vi "Unit Test.vi"() -> ()   [LabVIEW 2019, in "UIs.lvlib"]
uses:
  UIs.lvlib
  User Event/Controls/UE Abort Action.ctl
  Image/Image.lvlib
  Camera/Andor/Andor.lvlib
  Laser/Coherent/Coherent.lvlib
  LED/LED.lvlib
  Motion/Allmotion/Allmotion.lvlib
  Initialize/Initialize.lvlib
panel:
  in  "Laser":bool
  out "Motion":bool
  out "LED":bool
  out "Laser":bool
  out "Camera":bool
  in  "Open":bool
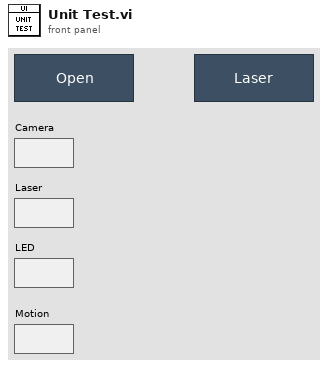
[diagram p1: front panel]
types:
  T1 = typedef "UE Abort Action.ctl" = enum16{"Create", "Get", "Destroy"}
  T2 = typedef "Andor.lvlib/SEQ Data.ctl" = cluster{"Initialize Sucess?":bool, "Image Ref":T3, "VI Refnum":refnum<vi>}
  T3 = typedef "IMAQ Image.ctl" = refnum<image>
  T4 = typedef "Coherent.lvlib/SEQ Data.ctl" = cluster{"Initialize Success?":bool, "VI Refnum":refnum<vi>}
  T5 = typedef "LED.lvlib/SEQ Data.ctl" = cluster{"Initialize Sucess?":bool, "BL2 Regulator":dbl, "BL1 Regulator":dbl, "Blood Sensor 1":dbl, "Blood Sensor 2":dbl, "Air Pressure Sensor":dbl, "Force Snesor 1":u32, "Force Snesor 2":u32, "VI Refnum":refnum<vi>}
  T6 = typedef "Allmotion.lvlib/SEQ Data.ctl" = cluster{"Position":i32[], "Arrived?":bool, "VISA name":refnum<visa-resource-name>, "Initialize Done?":bool, "State":string, "VI Refnum":refnum<vi>, "Dichroic Position":string[]}
  T7 = typedef "Initialize.lvlib/SEQ Data.ctl" = cluster{"Folder Path":path}
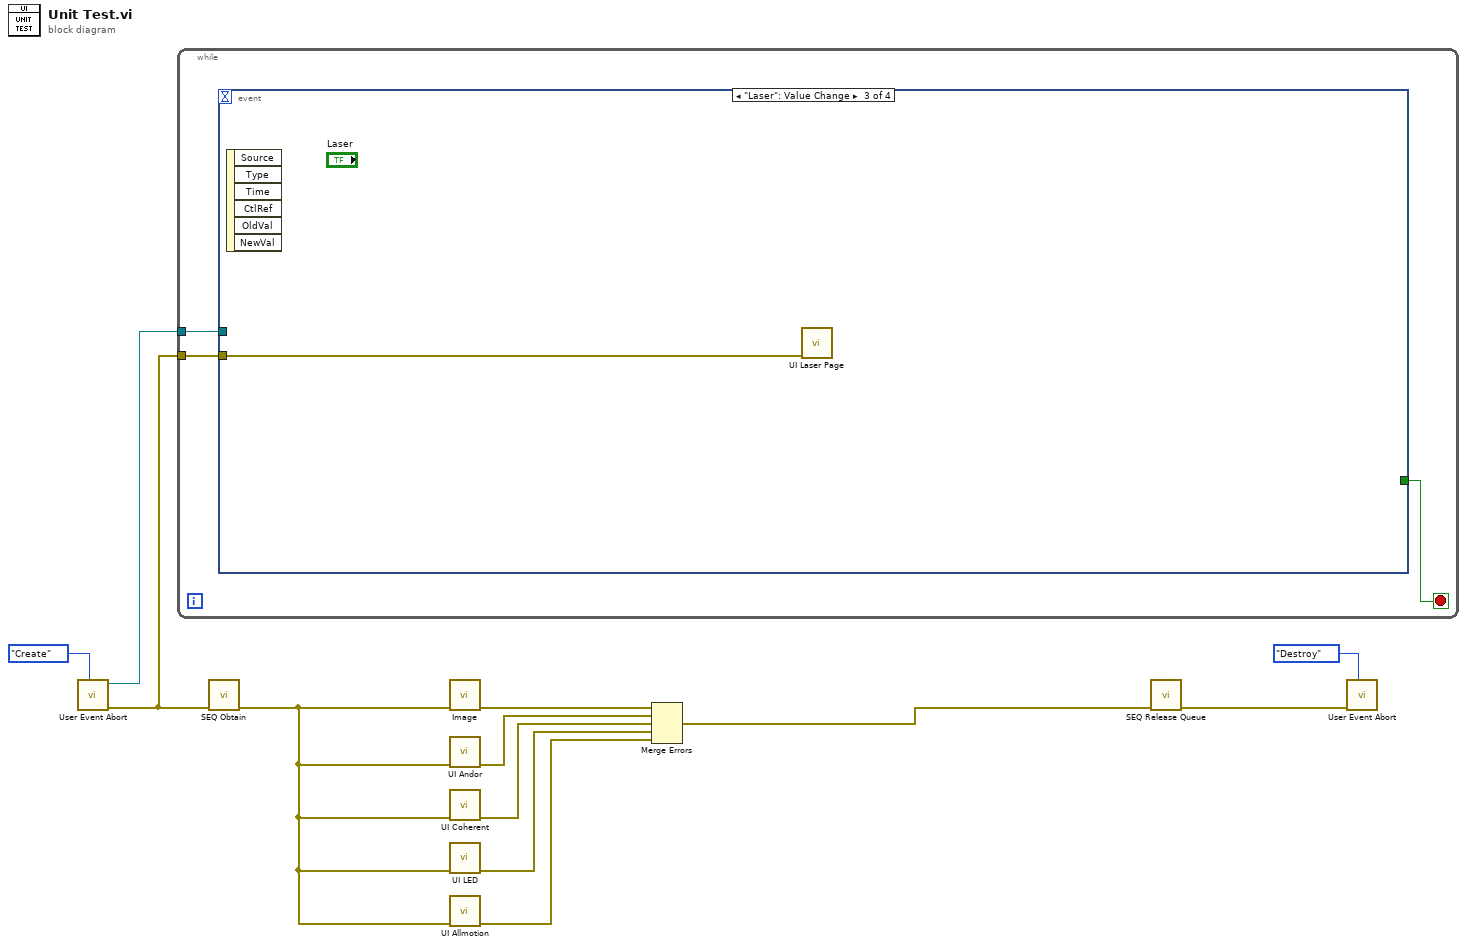
[diagram p0: block diagram]
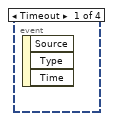
[diagram p2: hidden frame]
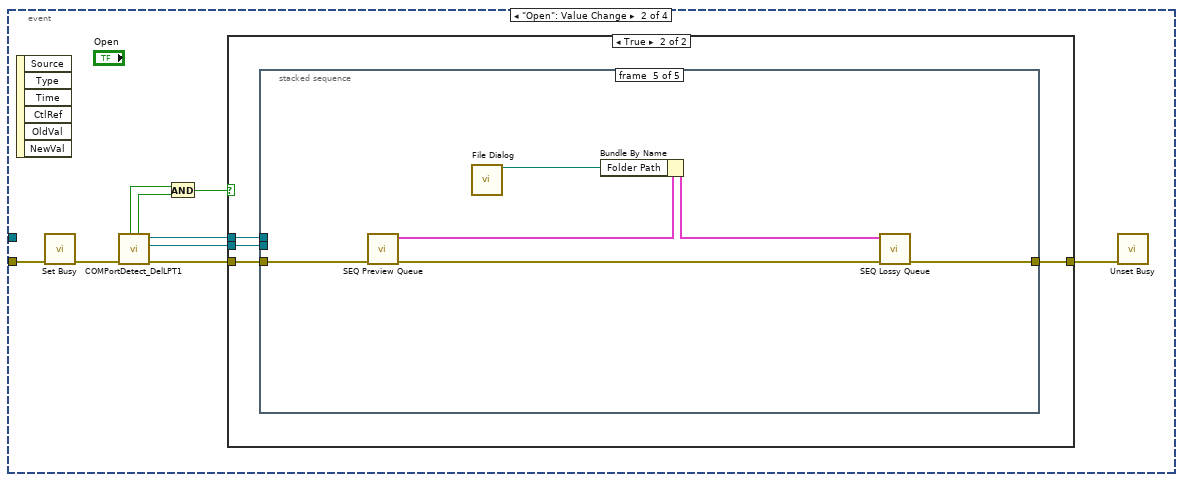
[diagram p3: hidden frame]
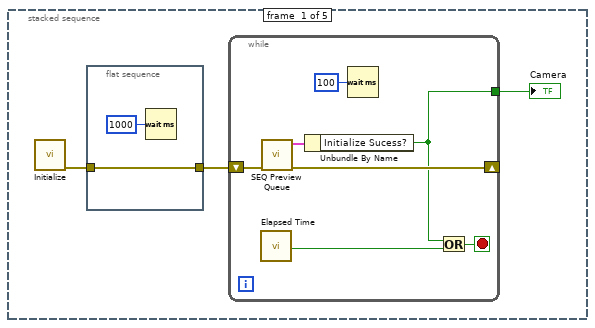
[diagram p5: hidden frame]
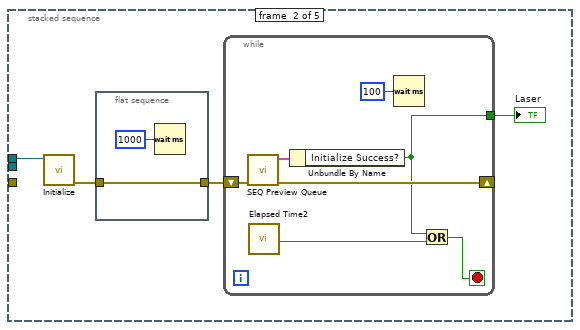
[diagram p6: hidden frame]
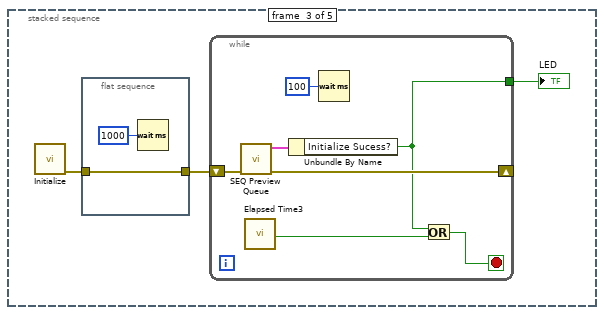
[diagram p7: hidden frame]
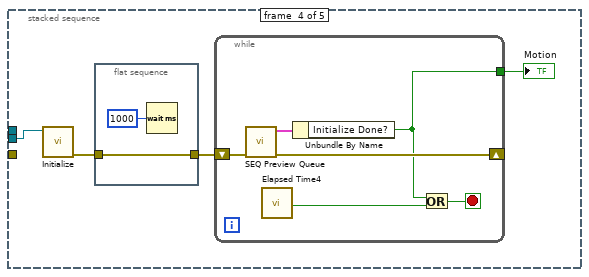
[diagram p8: hidden frame]
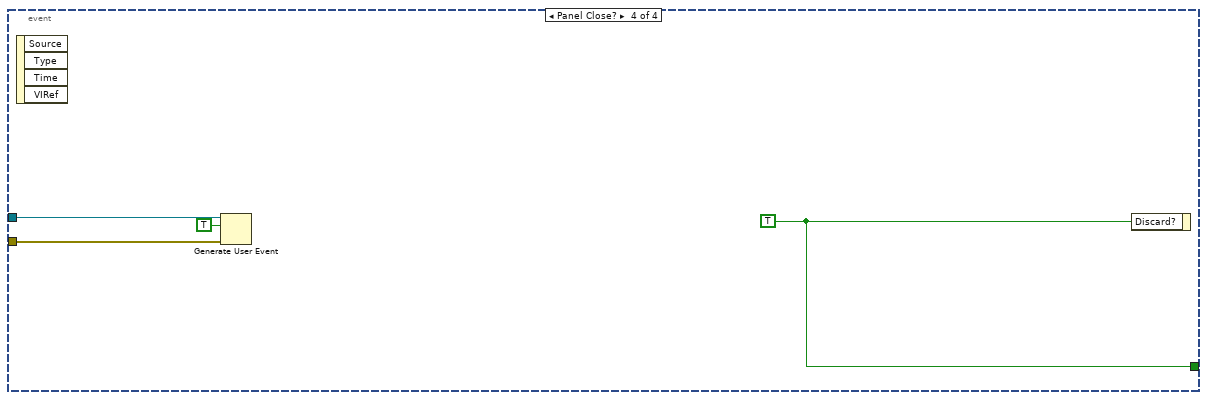
[diagram p9: hidden frame]
diagram:
  n1 = call "User Event Abort.vi"("Action"=UE_Abort_Action."Create") -> ("Error Out"=w2:errorcluster, "User Event Out"=w5:refnum<user-event>)  [unwired: 9 in]
  n2 = while {
    tunnel: w5 -> [w15]
    tunnel: w2 -> [w13]
    stop <- w14 stop-if-true
    n3 = event shown="[2] \"Laser\": Value Change" {
      selector: _ -> [_ _ _ _]
      dyn-events: _ -> [_ _ _ _]
      timeout: _ -> [_ _ _ _]
      tunnel: w15 -> [_ _ _ w88]
      tunnel: [_ _ _ w89] -> w14
      tunnel: w13 -> [_ w24 w85 w87]
      event Timeout {
        n4 = event-data() -> ()  [unwired: 1 in, 3 out]
      }
      event "Open": Value Change {
        n5 = event-data() -> ()  [unwired: 1 in, 6 out]
        n6 = call <vilib>:"Set Busy.vi"("error in (no error)"=w24) -> ("error out"=w22:errorcluster)  [unwired: 9 in, 1 out]
        n7 = call "COMPortDetect_DelLPT1.vi"("error in"=w22) -> ("error out"=w21:errorcluster, "VISA motion"=w16:refnum<visa-resource-name>, "VISA laser"=w17:refnum<visa-resource-name>, "Motion Find?"=w19:bool, "Laser Find?"=w20:bool)  [unwired: 6 in]
        n8 = And(x=w20, y=w19) -> (x .and. y?=w18:bool)
        n9 = case shown="True" w18 {
          tunnel: w21 -> [w25 w29]
          tunnel: [w25 w28] -> w23
          tunnel: w17 -> [_ w27]
          tunnel: w16 -> [_ w26]
          frame False {
          }
          frame True {
            n10 = stacked-sequence {
              tunnel: w29 -> [_ _ _ _ w84]
              tunnel: [_ _ _ _ w82] -> w28
              tunnel: w27 -> [_ w42 _ _ _]
              tunnel: w26 -> [_ _ _ w67 _]
              frame #0 {
                n11 = call "Initialize.vi"() -> ("Error Out"=w32:errorcluster)  [unwired: 11 in]
                n12 = flat-sequence {
                  tunnel: w32 -> [w40]
                  tunnel: [w40] -> w31
                  frame #0 {
                    n13 = Wait (ms)(milliseconds to wait=u32 1000) -> ()  [unwired: 1 out]
                  }
                }
                n14 = while {
                  shift-right: [w34] -> _
                  shift-left: w31 -> [w38]
                  tunnel: [w33] -> w30
                  stop <- w36 stop-if-true
                  n15 = call "Elapsed Time"() -> ("Time has Elapsed"=w35:bool)  [unwired: 12 in, 7 out]
                  n16 = call "SEQ Preview Queue.vi"("error in"=w38) -> ("error out"=w34:errorcluster, "SEQ Data"=w37:T2)  [unwired: 9 in]
                  n17 = Unbundle By Name(w37) -> ("Initialize Sucess?"=w33:bool)
                  n18 = Wait (ms)(milliseconds to wait=u32 100) -> ()  [unwired: 1 out]
                  n19 = Or(x=w33, y=w35) -> (x .or. y?=w36:bool)
                }
                "Camera" <- w30
              }
              frame #1 {
                n20 = call "Initialize.vi"("VISA in"=w42) -> ("Error Out"=w45:errorcluster)  [unwired: 10 in]
                n21 = flat-sequence {
                  tunnel: w45 -> [w53]
                  tunnel: [w53] -> w44
                  frame #0 {
                    n22 = Wait (ms)(milliseconds to wait=u32 1000) -> ()  [unwired: 1 out]
                  }
                }
                n23 = while {
                  shift-right: [w47] -> _
                  shift-left: w44 -> [w52]
                  tunnel: [w46] -> w43
                  stop <- w48 stop-if-true
                  n24 = call "SEQ Preview Queue.vi"("error in"=w52) -> ("error out"=w47:errorcluster, "SEQ Data"=w51:T4)  [unwired: 9 in]
                  n25 = call "Elapsed Time2"() -> ("Time has Elapsed"=w49:bool)  [unwired: 12 in, 7 out]
                  n26 = Unbundle By Name(w51) -> ("Initialize Success?"=w46:bool)
                  n27 = Wait (ms)(milliseconds to wait=u32 100) -> ()  [unwired: 1 out]
                  n28 = Or(x=w46, y=w49) -> (x .or. y?=w48:bool)
                }
                "Laser" <- w43
              }
              frame #2 {
                n29 = call "Initialize.vi"() -> ("Error Out"=w57:errorcluster)  [unwired: 11 in]
                n30 = flat-sequence {
                  tunnel: w57 -> [w65]
                  tunnel: [w65] -> w56
                  frame #0 {
                    n31 = Wait (ms)(milliseconds to wait=u32 1000) -> ()  [unwired: 1 out]
                  }
                }
                n32 = while {
                  shift-right: [w62] -> _
                  shift-left: w56 -> [w64]
                  tunnel: [w58] -> w55
                  stop <- w59 stop-if-true
                  n33 = call "SEQ Preview Queue.vi"("error in"=w64) -> ("error out"=w62:errorcluster, "SEQ Data"=w61:T5)  [unwired: 9 in]
                  n34 = call "Elapsed Time3"() -> ("Time has Elapsed"=w60:bool)  [unwired: 12 in, 7 out]
                  n35 = Unbundle By Name(w61) -> ("Initialize Sucess?"=w58:bool)
                  n36 = Wait (ms)(milliseconds to wait=u32 100) -> ()  [unwired: 1 out]
                  n37 = Or(x=w58, y=w60) -> (x .or. y?=w59:bool)
                }
                "LED" <- w55
              }
              frame #3 {
                n38 = call "Initialize.vi"("VISA in"=w67) -> ("Error Out"=w70:errorcluster)  [unwired: 10 in]
                n39 = flat-sequence {
                  tunnel: w70 -> [w71]
                  tunnel: [w71] -> w69
                  frame #0 {
                    n40 = Wait (ms)(milliseconds to wait=u32 1000) -> ()  [unwired: 1 out]
                  }
                }
                n41 = while {
                  shift-right: [w75] -> _
                  shift-left: w69 -> [w78]
                  tunnel: [w73] -> w68
                  stop <- w76 stop-if-true
                  n42 = call "SEQ Preview Queue.vi"("error in"=w78) -> ("error out"=w75:errorcluster, "SEQ Data"=w77:T6)  [unwired: 9 in]
                  n43 = call "Elapsed Time4"() -> ("Time has Elapsed"=w74:bool)  [unwired: 12 in, 7 out]
                  n44 = Unbundle By Name(w77) -> ("Initialize Done?"=w73:bool)
                  n45 = Or(x=w73, y=w74) -> (x .or. y?=w76:bool)
                }
                "Motion" <- w68
              }
              frame #4 {
                n46 = call "SEQ Preview Queue.vi"("error in"=w84) -> ("error out"=w83:errorcluster, "SEQ Data"=w81:T7)  [unwired: 9 in]
                n47 = call "File Dialog"() -> ("selected path"=w79:path)  [unwired: 12 in, 3 out]
                n48 = Bundle By Name(cluster=w81, "Folder Path"=w79) -> (w80:T7)
                n49 = call "SEQ Lossy Queue.vi"("error in"=w83, "SEQ Data"=w80) -> ("error out"=w82:errorcluster)  [unwired: 9 in]
              }
            }
          }
        }
        n50 = call <vilib>:"Unset Busy.vi"("error in (no error)"=w23) -> ()  [unwired: 10 in, 1 out]
      }
      event "Laser": Value Change {
        n51 = event-data() -> ()  [unwired: 1 in, 6 out]
        n52 = call "UI Laser Page.vi"("error in"=w85) -> ()  [unwired: 10 in, 1 out]
      }
      event Panel Close? {
        w89 = TRUE ("Discard?")
        n53 = event-data() -> ()  [unwired: 1 in, 4 out]
        n54 = Generate User Event(user event=w88, event data cluster=TRUE ("event data"), error in=w87) -> ()  [unwired: 1 in, 2 out]
        n55 = event-data("Discard?"=w89) -> ()  [unwired: 1 in, 1 out]
      }
    }
  }
  n56 = call "SEQ Obtain.vi"("error in"=w2) -> ("error out"=w1:errorcluster)  [unwired: 9 in, 1 out]
  n57 = call "Image.vi"("error in"=w1) -> ("error out"=w12:errorcluster)  [unwired: 10 in]
  n58 = call "UI Andor.vi"("error in"=w1) -> ("error out"=w11:errorcluster)  [unwired: 10 in]
  n59 = call "UI Coherent.vi"("error in"=w1) -> ("error out"=w10:errorcluster)  [unwired: 10 in]
  n60 = call "UI LED.vi"("error in"=w1) -> ("error out"=w9:errorcluster)  [unwired: 10 in]
  n61 = call "UI Allmotion.vi"("error in"=w1) -> ("error out"=w8:errorcluster)  [unwired: 10 in]
  n62 = Merge Errors(w12, w11, w10, w9, w8) -> (w4:errorcluster)
  n63 = call "SEQ Release Queue.vi"("error in"=w4) -> ("error out"=w3:errorcluster)  [unwired: 10 in]
  n64 = call "User Event Abort.vi"("Action"=UE_Abort_Action."Destroy", "Error In"=w3) -> ()  [unwired: 8 in, 2 out]
